vi "SP Sort Adapters by Order.vi"(3 "Port":i8, 4 "Adapters":T1[](array[typedef])) -> (1 "Sorted Adapters":T1[](array[typedef]))   [LabVIEW 2011]
uses:
  TypeDefs/SP Adapter.ctl
  TypeDefs/SP Data.ctl
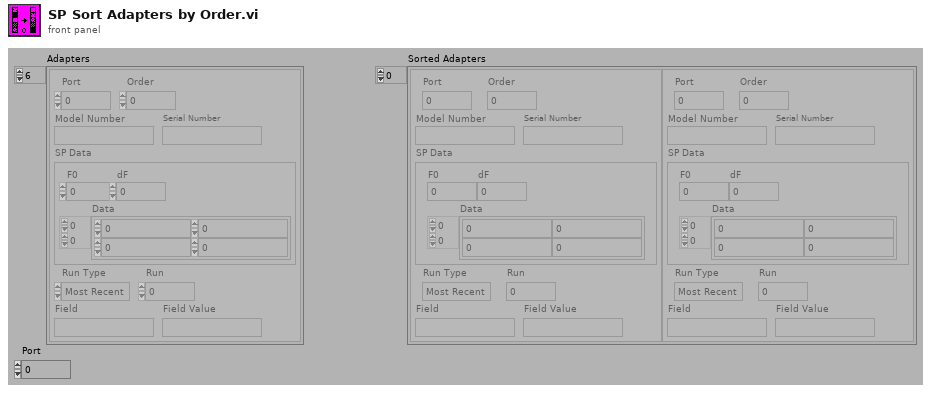
[diagram p1: front panel]
types:
  T1 = typedef "SP Adapter.ctl" = cluster{"Port":i8, "Order":i8, "Model Number":string, "Serial Number":string, "SP Data":T2, "Run Type":enum16{"Most Recent", "Run #", "Match Field"}, "Run":i32, "Field":string, "Field Value":string}
  T2 = typedef "SP Data.ctl" = cluster{"F0":dbl, "dF":dbl, "Data":cdb[][]}
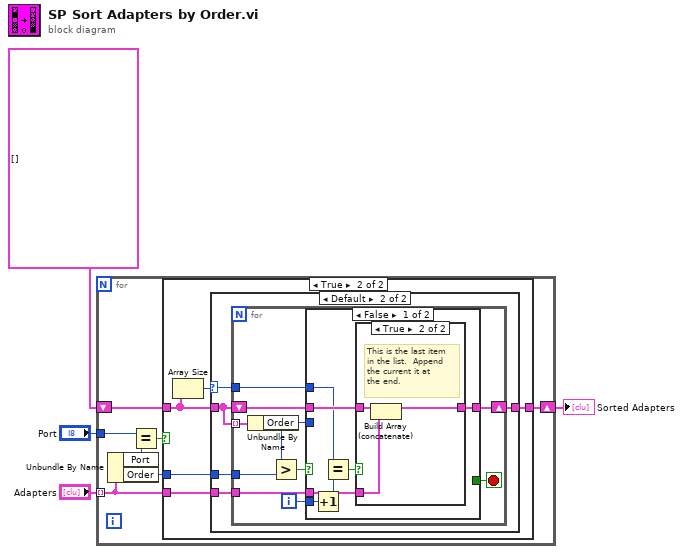
[diagram p0: block diagram]
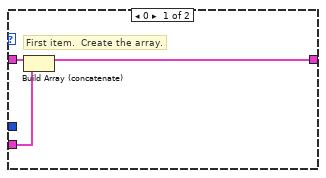
[diagram p3: hidden frame]
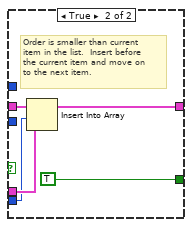
[diagram p5: hidden frame]
diagram:
  n1 = for {
    tunnel: "Adapters" -> [w6] mode=indexing
    tunnel: "Port" -> [w11]
    shift-right: [w7] -> w1
    shift-left: T1[] [] ("Adapters") -> [w8]
    n2 = Unbundle By Name(w6) -> ("Port"=w10:i8, "Order"=w5:i8)
    n3 = Equal?(x=w11, y=w10) -> (x = y?=w9:bool)
    n4 = case shown="True" w9 {
      tunnel: w8 -> [w12 w14]
      tunnel: [w12 w15] -> w7
      tunnel: w6 -> [_ w16]
      tunnel: w5 -> [_ w17]
      frame False {
      }
      frame True {
        n5 = Array Size(array=w14) -> (size(s)=w13:i32)
        n6 = case shown="Default" w13 {
          selector: w13 -> [_ w21]
          tunnel: w17 -> [_ w25]
          tunnel: w16 -> [w19 w24]
          tunnel: [w18 w23] -> w15
          tunnel: w14 -> [w20 w22]
          frame 0 {
            # "First item.  Create the array."
            n7 = Build Array (concatenate)(w20, w19) -> (w18:T1[])
          }
          frame Default {
            n8 = for {
              tunnel: w22 -> [w35] mode=indexing
              tunnel: w25 -> [w34]
              tunnel: w24 -> [w31]
              shift-right: [w29] -> w23
              shift-left: w22 -> [w30]
              tunnel: w21 -> [w26]
              i -> [w28]
              stop <- w27 stop-if-true
              n9 = Unbundle By Name(w35) -> ("Order"=w32:i8)
              n10 = Greater?(x=w32, y=w34) -> (0:w33:bool)
              n11 = case shown="False" w33 {
                tunnel: [w37 w51] -> w29
                tunnel: [_ TRUE] -> w27
                tunnel: w32 -> [_ _]
                tunnel: w31 -> [w39 w48]
                tunnel: w30 -> [w38 w49]
                tunnel: w28 -> [w41 w47]
                tunnel: w26 -> [w36 _]
                frame False {
                  n12 = Increment(x=w41) -> (x+1=w42:i32)
                  n13 = Equal?(x=w36, y=w42) -> (x = y?=w40:bool)
                  n14 = case shown="True" w40 {
                    tunnel: w38 -> [w43 w46]
                    tunnel: w39 -> [_ w45]
                    tunnel: [w43 w44] -> w37
                    frame False {
                      # "Move on to the\nnext item and\ncheck again."
                    }
                    frame True {
                      # "This is the last item\nin the list.  Append\nthe current it at \nthe end."
                      n15 = Build Array (concatenate)(w46, w45) -> (w44:T1[])
                    }
                  }
                }
                frame True {
                  # "Order is smaller than current\nitem in the list.  Insert before\nthe current item and move on\nto the next item."
                  n16 = Insert Into Array(array=w49, index=w47, new element=w48) -> (w51:T1[])
                }
              }
            }
          }
        }
      }
    }
  }
  "Sorted Adapters" <- w1
